vi "ConfigureLevel.vi"(8 "error in (no error)":errorcluster, 10 "Threshold":T1=enum."INFO", 11 "Logger in":refnum<class "Logger.lvclass">) -> (0 "error out":errorcluster, 3 "Logger out":refnum<class "Logger.lvclass">)   [LabVIEW 2026, in "Lumberjack.lvlib" / "Logger.lvclass"]
doc: "Changes the running global severity threshold.\nResolves the logger and sends a SetGlobalThresholdMsg carrying Threshold to the LogManager, which updates the global gate and re-posts the Snapshot so stage-1 gating uses the new level. No-op passthrough if no logger resolves.\nLumberjack.lvlib, Logger.lvclass, public."
uses:
  Logger.lvclass
  TypeDefs/Severity.ctl
  Logger.lvclass/Logger.ctl
  <vilib>/ActorFramework/Message Enqueuer/Message Enqueuer.lvclass
  Core/Messages/SetGlobalThresholdMsg.lvclass/SetGlobalThresholdMsg.lvclass
  Lumberjack.lvlib
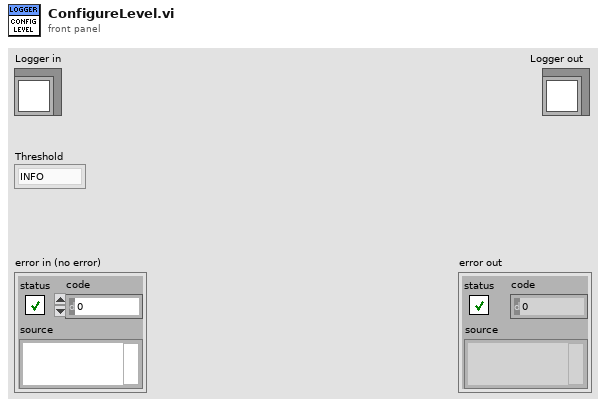
[diagram p1: front panel]
types:
  T1 = typedef "Lumberjack.lvlib/Severity.ctl" = enum16{"OFF", "FATAL", "ERROR", "WARN", "INFO", "DEBUG", "TRACE", "ALL"}
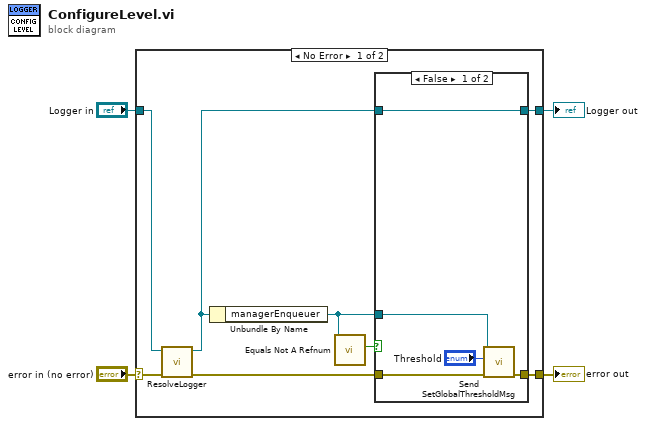
[diagram p0: block diagram]
diagram:
  n1 = case shown="No Error" "error in (no error)" {
    selector: "error in (no error)" -> [w12 w21]
    tunnel: [w10 w21] -> w3
    tunnel: [w8 w20] -> w1
    tunnel: "Logger in" -> [w9 w20]
    frame No Error {
      n2 = call "ResolveLogger.vi"("error in (no error)"=w12, "Logger in"=w9) -> ("error out"=w11:errorcluster, "Logger out"=w7:refnum<class "Logger.lvclass">)  [unwired: 8 in]
      n3 = Unbundle By Name(w7) -> ("managerEnqueuer"=w5:refnum<class "Message Enqueuer.lvclass">)
      n4 = call <vilib>:"Equals Not A Refnum.vi"("Message Enqueuer"=w5) -> ("Not a refnum?"=w6:bool)  [unwired: 10 in]
      n5 = case shown="False" w6 {
        tunnel: w11 -> [w17 w19]
        tunnel: [w16 w19] -> w10
        tunnel: [w15 w18] -> w8
        tunnel: w7 -> [w15 w18]
        tunnel: w5 -> [w14 _]
        frame False {
          n6 = call "Send SetGlobalThresholdMsg.vi"("error in (no error)"=w17, "Threshold"="Threshold", "Enqueuer in"=w14) -> ("error out"=w16:errorcluster)  [unwired: 7 in, 1 out]
        }
        frame True {
        }
      }
    }
    frame Error {
    }
  }
  "error out" <- w3
  "Logger out" <- w1
